vi "기능적 글로벌 변수 실습.vi"() -> ()   [LabVIEW 2020]
panel:
  in  "정지 2":bool
  in  "정지":bool
  out "웨이브폼 차트 2":dbl(graph)
  out "웨이브폼 차트":dbl(graph)
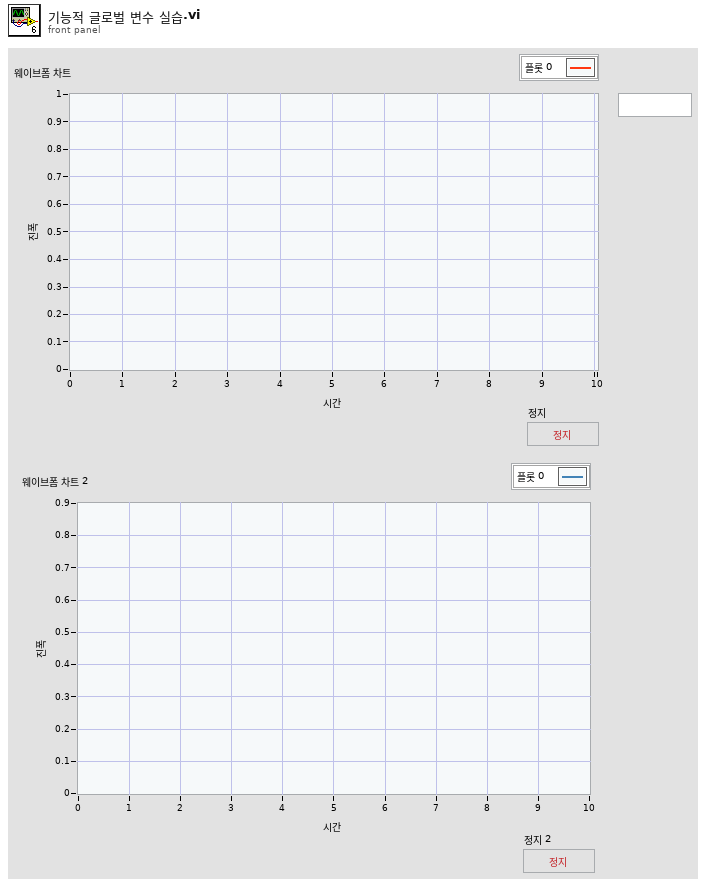
[diagram p1: front panel]
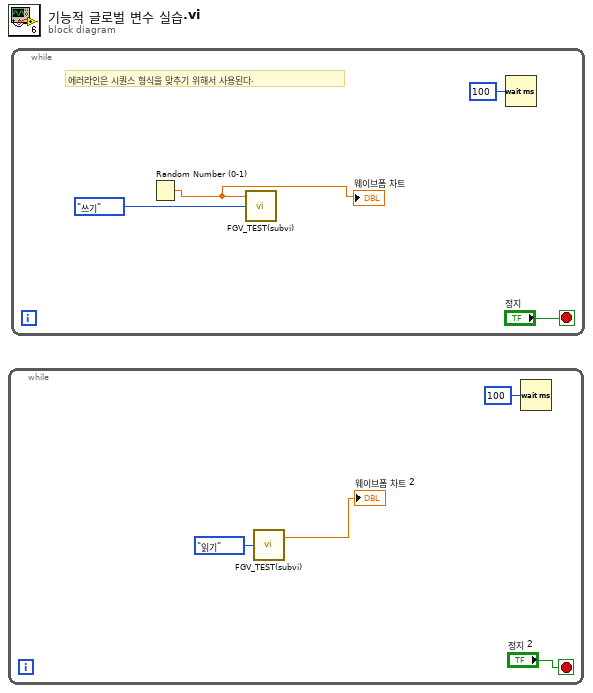
[diagram p0: block diagram]
diagram:
  n1 = while {
    stop <- "정지 2" stop-if-true
    n2 = call "FGV_TEST(subvi).vi"("상태컨트롤"=enum16{"초기화", "읽기", "쓰기"}."읽기") -> ("OUT"=→"웨이브폼 차트 2":dbl)  [unwired: 2 in, 1 out]
    n3 = Wait (ms)(milliseconds to wait=u32 100 ("대기 시간 (ms)")) -> ()  [unwired: 1 out]
  }
  n4 = while {
    stop <- "정지" stop-if-true
    # "에러라인은 시퀀스 형식을 맞추기 위해서 사용된다."
    n5 = Random Number (0-1)() -> (number: 0 to 1=w6:dbl)
    "웨이브폼 차트" <- w6
    n6 = call "FGV_TEST(subvi).vi"("상태컨트롤"=enum16{"초기화", "읽기", "쓰기"}."쓰기", "IN"=w6) -> ()  [unwired: 1 in, 2 out]
    n7 = Wait (ms)(milliseconds to wait=u32 100 ("대기 시간 (ms)")) -> ()  [unwired: 1 out]
  }
